vi "Create from SFTP.vi"(8 "Error In":errorcluster, 11 "SFTP In":refnum<class "SFTP.lvclass">) -> (0 "Error Out":errorcluster, 2 "SFTP Attributes":refnum<class "SFTP Attributes.lvclass">, 3 "SFTP Out":refnum<class "SFTP.lvclass">)   [LabVIEW 2018, in "Toolkit.lvlib" / "SFTP Attributes.lvclass"]
doc: "Passes through the SFTP object but obtains the SSH context for the SFTP object to create a new SFTP Attributes object."
uses:
  SFTP Attributes.lvclass
  SFTP/SFTP.lvclass
  SFTP/SFTP.lvclass/SFTP.ctl
  Session/Session.lvclass/Session.ctl
  SSH/SSH.lvclass
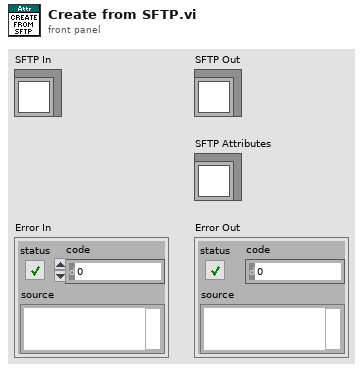
[diagram p1: front panel]
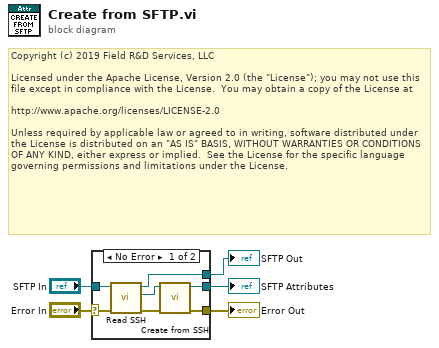
[diagram p0: block diagram]
diagram:
  # "Copyright (c) 2019 Field R&D Services, LLC\n\nLicensed under the Apache License, Version 2.0 (the \"License\"); you may not use this file except in compliance with the License.  You may obtain a copy of the License at\n\nhttp://www.apache.org/licenses/LICENSE-2.0\n\nUnless required by applicable law or agreed to in writing, software distributed under the License is distributed on an \"AS IS\" BASIS, WITHOUT WARRANTIES OR CONDITIONS OF ANY KIND, either express or implied.  See the License for the specific language governing permissions and limitations under the License."
  n1 = case shown="No Error" "Error In" {
    selector: "Error In" -> [w10 w14]
    tunnel: [w11 w14] -> w4
    tunnel: [w12 _] -> w3
    tunnel: "SFTP In" -> [w9 w13]
    tunnel: [w6 w13] -> w1
    frame No Error {
      n2 = call "Read SSH.vi"("Error In"=w10, "SFTP In"=w9) -> ("Erorr Out"=w7:errorcluster, "SSH"=w8:refnum<class "SSH.lvclass">, "SFTP Out"=w6:refnum<class "SFTP.lvclass">)  [unwired: 7 in]
      n3 = call "Create from SSH.vi"("Error In"=w7, "SSH"=w8) -> ("Error Out"=w11:errorcluster, "SFTP Attributes"=w12:refnum<class "SFTP Attributes.lvclass">)  [unwired: 8 in]
    }
    frame Error {
    }
  }
  "Error Out" <- w4
  "SFTP Attributes" <- w3
  "SFTP Out" <- w1
